vi "LDH2_Inline_scan_trigger_out_v6_Multisite_CLC.vi"(0 "Acquisition Height":u32, 5 "Loop Num":i32, 9 "Master Ctr Task In":refnum<k21>, 11 "error in":errorcluster, 12 "Stop (F)":bool) -> (1 "Master Ctr Task Out":refnum<k21>, 3 "Acquired Buffer Number":u32, 4 "Image Pixels (I16)":i16[][](array[numeric]), 6 "Image Out":T1(plugin-control), 10 "Frame Rate":dbl, 13 "First frm":u32, 14 "Stopped":bool, 15 "error out":errorcluster)   [LabVIEW 2019]
doc: "Creates, and edits acquisitions using the NI Vision Acquisition Express VI.\n\nThe NI Vision Acquisition Wizard is launched by placing the Express VI on the block diagram. Select an acquisition source and configure an acquisition using NI-IMAQ, NI-IMAQdx, or simulate an acquisition by reading an AVI or image files from a folder. After an acquisition is configured, select controls and indicators to be able to programmatically set in LabVIEW. Double-click the Vision Acquisition Express VI to edit the acquisition.\n\nNote: Any images created by the Express VI need to be disposed after use. Use the IMAQ Dispose.vi to cleanup the images output by the Express VI when they are no longer needed."
panel:
  in  "Pulse Delay":dbl
  in  "Pulse Width":dbl
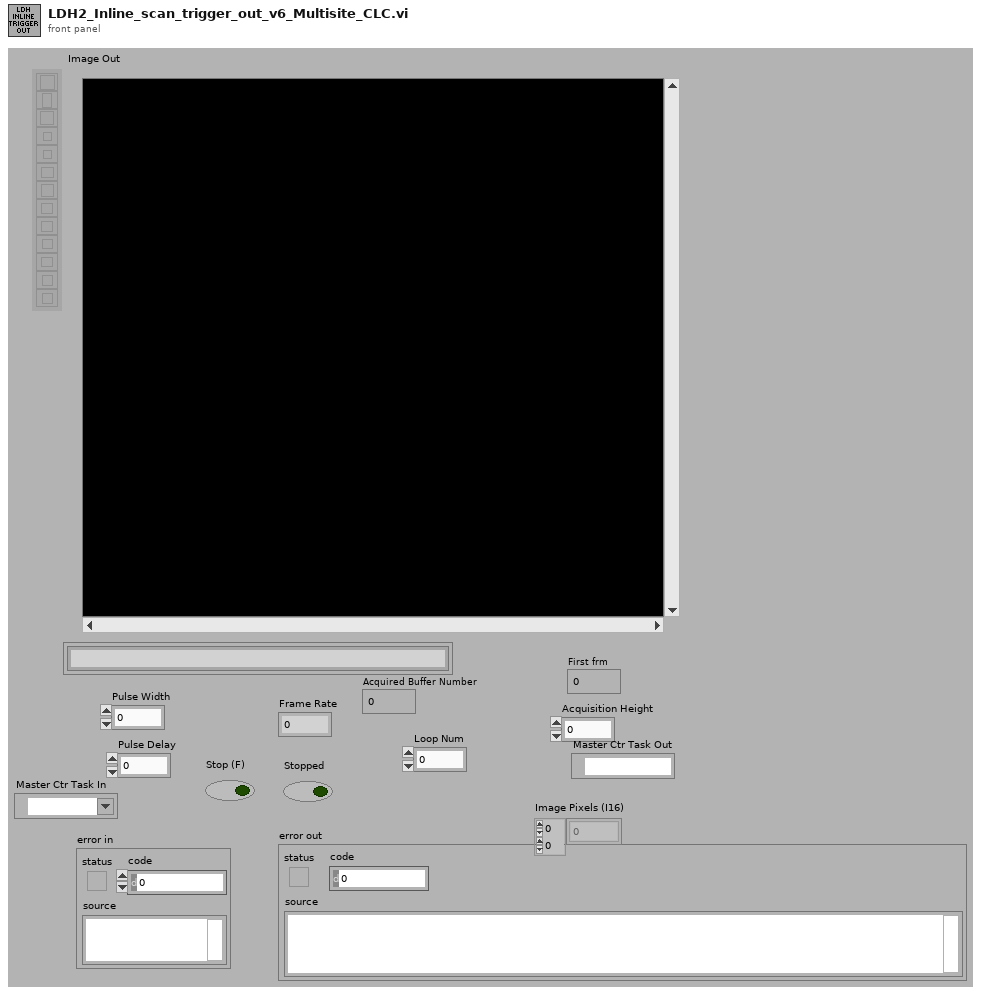
[diagram p1: front panel]
types:
  T1 = typedef "IMAQ Image.ctl" = refnum<image>
  T2 = cluster{"Pulse Delay":dbl, "Pulse Width":dbl, "Pulse Polarity":enum16{"High True ", "Low True"}, "Units":enum16{"Seconds", "Scaled Encoder Counts"}}
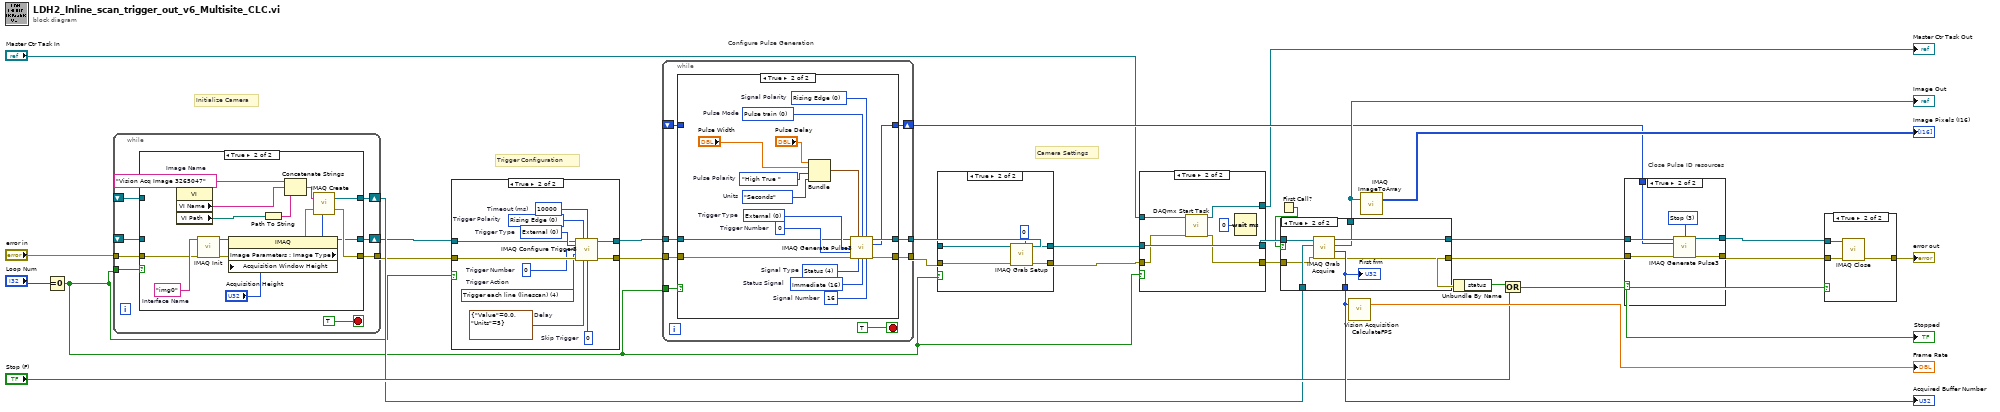
[diagram p0: block diagram]
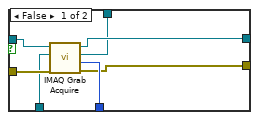
[diagram p2: hidden frame]
diagram:
  # "Camera Settings"
  # "Initialize Camera"
  # "Trigger Configuration"
  # "Close Pulse ID resources"
  # "Configure Pulse Generation"
  n1 = Equal To 0?(x="Loop Num") -> (x = 0?=w4:bool)
  n2 = while "While Loop_template0_template1" {
    tunnel: w4 -> [w38]
    tunnel: [w35] -> w14
    tunnel: "error in" -> [w34]
    shift-right: [w32] -> w25
    shift-left: _ -> [w31]
    shift-right: [w37] -> w15
    shift-left: _ -> [w36]
    stop <- TRUE ("_template0_template1") stop-if-true
    n3 = case "Case Structure_template0_template1" shown="True" w38 {
      tunnel: [w41 w43] -> w37
      tunnel: w36 -> [w41 _]
      tunnel: [w40 w44] -> w35
      tunnel: w34 -> [w40 w52]
      tunnel: [w39 w54] -> w32
      tunnel: w31 -> [w39 _]
      frame False {
      }
      frame True {
        w53 = "img0"  # Interface Name
        w48 = "Vision Acq Image 3265047"  # Image Name
        n4 = property class="VI"() -> ("VI Name"=w50:string, "VI Path"=w51:path)  [unwired: 2 in, 2 out]
        n5 = call <vilib>:"IMAQ Init.vi"("error in (no error)"=w52, "Interface Name"=w53) -> ("error out"=w45:errorcluster, "IMAQ Session Out"=w46:refnum<k11>)  [unwired: 8 out]
        n6 = property class="IMAQ"(reference=w46, error in=w45, "Acquisition Window Height"="Acquisition Height") -> (reference out=w43:refnum<k11>, error out=w56:errorcluster, "Image Parameters : Image Type"=w55:u32)
        n7 = Path To String(path=w51) -> (string=w49:string)
        n8 = Concatenate Strings(w48, w50, w49) -> (w47:string)
        n9 = call "IMAQ Create"("Image Name"=w47, "Image Type"=w55, "error in (no error)"=w56) -> ("New Image"=w54:T1, "error out"=w44:errorcluster)  [unwired: 1 in, 1 out]
      }
    }
  }
  n10 = case "Case Structure_template0_template1" shown="True" w4 {
    tunnel: w15 -> [w58 w66]
    tunnel: w14 -> [w57 w65]
    tunnel: [w58 w64] -> w13
    tunnel: [w57 w63] -> w12
    frame False {
    }
    frame True {
      w59 = cluster{"Value":dbl, "Units":u32} {"Value"=0.0, "Units"=5}  # Delay
      w62 = u32 10000  # Timeout (ms)
      w67 = u32 0 items=["Rising Edge", "Falling Edge"]  # Trigger Polarity
      w69 = u32 0  # Skip Trigger
      w60 = u32 4 items=["Disabled", "Trigger start of acquisition", "Trigger start of each buffer list", "Trigger each buffer", "Trigger each line (linescan)", "Trigger end of acquisition"]  # Trigger Action
      w61 = u32 0  # Trigger Number
      w68 = u32 0 items=["External"=0, "RTSI"=1, "ISO In"=2, "Scaled Encoder"=5]  # Trigger Type
      n11 = call <vilib>:"IMAQ Configure Trigger3.vi"("IMAQ Session In"=w66, "Polarity"=w67, "Frame timeout (ms)"=w62, "Type"=w68, "Line Number"=w61, "Action"=w60, "error in (no error)"=w65, "Delay"=w59, "Skip trigger (linescan only)"=w69) -> ("IMAQ Session Out"=w64:refnum<k11>, "error out"=w63:errorcluster)  [unwired: 5 out]
    }
  }
  n12 = while {
    tunnel: w4 -> [w77]
    tunnel: w13 -> [w76]
    tunnel: [w75] -> w10
    tunnel: [w74] -> w11
    tunnel: w12 -> [w73]
    shift-right: [w72] -> w9
    shift-left: _ -> [w70]
    stop <- TRUE stop-if-true
    n13 = case "Case Structure_template0_template1" shown="True" w77 {
      tunnel: w76 -> [w80 w88]
      tunnel: w73 -> [w79 w85]
      tunnel: [w80 w87] -> w75
      tunnel: [w79 w86] -> w74
      tunnel: [w78 w84] -> w72
      tunnel: w70 -> [w78 _]
      frame False {
      }
      frame True {
        w91 = enum16{"High True ", "Low True"}."High True "  # Pulse Polarity
        w92 = enum16{"Seconds", "Scaled Encoder Counts"}."Seconds"  # Units
        w89 = u32 0 items=["Rising Edge", "Falling Edge"]  # Signal Polarity
        w94 = u32 0  # Trigger Number
        w93 = u32 0 items=["External"=0, "RTSI"=1, "ISO Out"=3]  # Trigger Type
        w97 = u32 16  # Signal Number
        w96 = u32 16 items=["Acquisition in progress"=15, "Acquisition done"=8, "Horizontal Synchronization Signal"=18, "Vertical Synchronization Signal"=19, "Frame start"=9, "Frame done"=10, "Immediate"=16]  # Status Signal
        w95 = u32 4 items=["External"=0, "RTSI "=1, "ISO In"=2, "Status"=4]  # Signal Type
        w90 = u32 0 items=["Pulse train", "Single pulse", "Rearmed pulse", "Stop"]  # Pulse Mode
        n14 = Bundle("Pulse Delay"="Pulse Delay", "Pulse Width"="Pulse Width", "Pulse Polarity"=w91, "Units"=w92) -> (w83:T2)  [unwired: 1 out]
        n15 = call <vilib>:"IMAQ Generate Pulse3.vi"("IMAQ Session In"=w88, "Pulse Parameters"=w83, "Pulse Mode"=w90, "Signal polarity"=w89, "Trigger Type"=w93, "Trigger Number"=w94, "error in (no error)"=w85, "Signal Type"=w95, "Status Signal"=w96, "Signal Number"=w97) -> ("IMAQ Session Out"=w87:refnum<k11>, "Pulse ID Out"=w84:u32, "error out"=w86:errorcluster)  [unwired: 1 in, 2 out]
      }
    }
  }
  n16 = case shown="True" w4 {
    tunnel: w10 -> [w99 w103]
    tunnel: [w99 w102] -> w6
    tunnel: [w98 w101] -> w5
    tunnel: w11 -> [w98 w100]
    frame False {
    }
    frame True {
      n17 = call <vilib>:"IMAQ Grab Setup.vi"("Channel"=0, "error in (no error)"=w100, "IMAQ Session In"=w103) -> ("error out"=w101:errorcluster, "IMAQ Session Out"=w102:refnum<k11>)  [unwired: 7 out]
    }
  }
  n18 = case shown="True" w4 {
    tunnel: w6 -> [w107 w113]
    tunnel: [w107 w113] -> w8
    tunnel: [w106 w111] -> w7
    tunnel: w5 -> [w106 w112]
    tunnel: "Master Ctr Task In" -> [w105 w110]
    tunnel: [w105 w109] -> w2
    frame False {
    }
    frame True {
      n19 = call <vilib>:"DAQmx Start Task.vi"("task/channels in"=w110, "error in"=w112) -> ("task out"=w109:refnum<k21>, "error out"=w111:errorcluster)  [unwired: 12 in]
      n20 = Wait (ms)(milliseconds to wait=u32 0) -> ()  [unwired: 1 out]
    }
  }
  "Master Ctr Task Out" <- w2
  n21 = First Call?() -> (First Call?: T/F=w1:bool)
  n22 = case shown="True" w1 {
    tunnel: [w115 w127] -> w29
    tunnel: w25 -> [w118 w126]
    tunnel: [w114 w125] -> w24
    tunnel: [w117 w124] -> w22
    tunnel: [w116 w123] -> w18
    tunnel: w8 -> [w120 w122]
    tunnel: w7 -> [w119 w121]
    frame False {
      n23 = call <vilib>:"IMAQ Grab Acquire.vi"("error in (no error)"=w119, "Image In"=w118, "IMAQ Session In"=w120) -> ("error out"=w114:errorcluster, "Acquired Buffer Number"=w115:u32, "Image Out"=w116:T1, "IMAQ Session Out"=w117:refnum<k11>)  [unwired: 1 in, 4 out]
    }
    frame True {
      n24 = call <vilib>:"IMAQ Grab Acquire.vi"("error in (no error)"=w121, "Image In"=w126, "IMAQ Session In"=w122) -> ("error out"=w125:errorcluster, "Acquired Buffer Number"=w127:u32, "Image Out"=w123:T1, "IMAQ Session Out"=w124:refnum<k11>)  [unwired: 1 in, 4 out]
      "First frm" <- w127
    }
  }
  "Image Out" <- w18
  "Acquired Buffer Number" <- w29
  n25 = call <vilib>:"Vision Acquisition CalculateFPS.vi"("buffer number"=w29) -> ("acquired FPS"=→"Frame Rate":dbl)  [unwired: 2 out]
  n26 = call "IMAQ ImageToArray"("Image"=w18) -> ("Image Pixels (I16)"=→"Image Pixels (I16)":i16[][])  [unwired: 3 in, 4 out]
  n27 = Unbundle By Name(w24) -> ("status"=w27:bool)
  n28 = Or(x=w27, y="Stop (F)") -> (x .or. y?=w20:bool)
  "Stopped" <- w20
  n29 = case shown="True" w20 {
    tunnel: [w129 w135] -> w21
    tunnel: [w128 w134] -> w23
    tunnel: w24 -> [w128 w133]
    tunnel: w22 -> [w129 w132]
    tunnel: w9 -> [_ w131]
    frame False {
    }
    frame True {
      w130 = u32 3 items=["Pulse train", "Single pulse", "Rearmed pulse", "Stop"] ("Pulse Mode")
      n30 = call <vilib>:"IMAQ Generate Pulse3.vi"("IMAQ Session In"=w132, "Pulse Mode"=w130, "Pulse ID In"=w131, "error in (no error)"=w133) -> ("IMAQ Session Out"=w135:refnum<k11>, "error out"=w134:errorcluster)  [unwired: 7 in, 3 out]
    }
  }
  n31 = case "Case Structure_template2" shown="True" w20 {
    tunnel: [w136 w139] -> w19
    tunnel: w21 -> [_ w137]
    tunnel: w23 -> [w136 w138]
    frame False {
    }
    frame True {
      n32 = call <vilib>:"IMAQ Close.vi"("error in (no error)"=w138, "IMAQ Session In"=w137) -> ("error out"=w139:errorcluster)  [unwired: 9 out]
    }
  }
  "error out" <- w19
